vi "MBmaster.vi_tom.vi"(0 "Register address (0)":u16 max=247 format="%.0x", 1 "Modbus address (1)":u8=1 max=247, 2 "port number":i32, 5 "No. of points (1)":u16 max=247, 7 "Setpoints (0)":dbl[](array[numeric]) max=247.0 format="%.2f", 9 "Set digitals":bool[](array[boolean]), 11 "error in (no error)":errorcluster, 12 "Decimal points (0)":u8[](array[numeric]) max=4, 13 "ModBus Function":T1(ring)=enum."03 Read output registers") -> (4 "String send to device":string, 6 "String received from device":string, 8 "Process values":dbl[](array[numeric]) max=247.0 format="%.2f", 10 "Digitals read":bool[](array[boolean]), 15 "error out":errorcluster)   [LabVIEW 2010]
doc: "VI let you communicatie via a serial inerface with Modbus instruments.\n\nPS. No error checking is done in this version; Error clusters only implemented for future use - Users might implement this for their own needs...\n\nThis VI is referenced to the Modicon Modbus Protocol as described in the Modicon Modbus Protocol Reference Guide PI-MBUS-300 rev. D\n\nThis VI is only tested with a Eurotherm T103 unit controller but should alse work with any other Modbus Instrument.\n\nMaarten van Bree\nAIR technical automation, the Netherlands\n\nmvbree@euronet.nl\ninfo@air.nl\nhttp://www.air.nl"
panel:
  out "Calculated CRC":u16 format="%.0x"
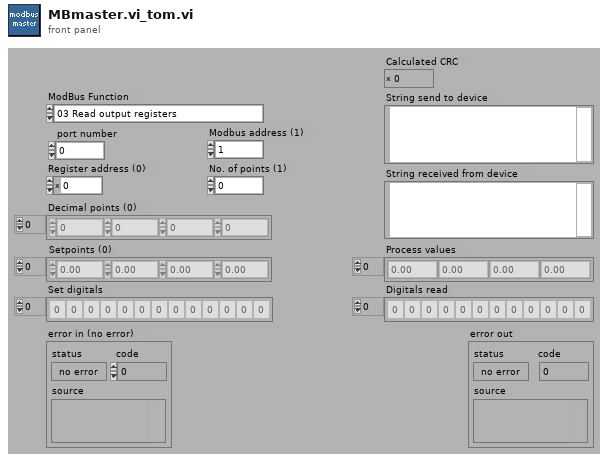
[diagram p1: front panel]
types:
  T1 = enum16{"01 Read digital output status", "02 Read digital input status", "03 Read output registers", "04 Read input registers", "05 Write single digital output", "06 Write single output register", "15 Write multiple digital outputs", "16 Write multiple output registers"}
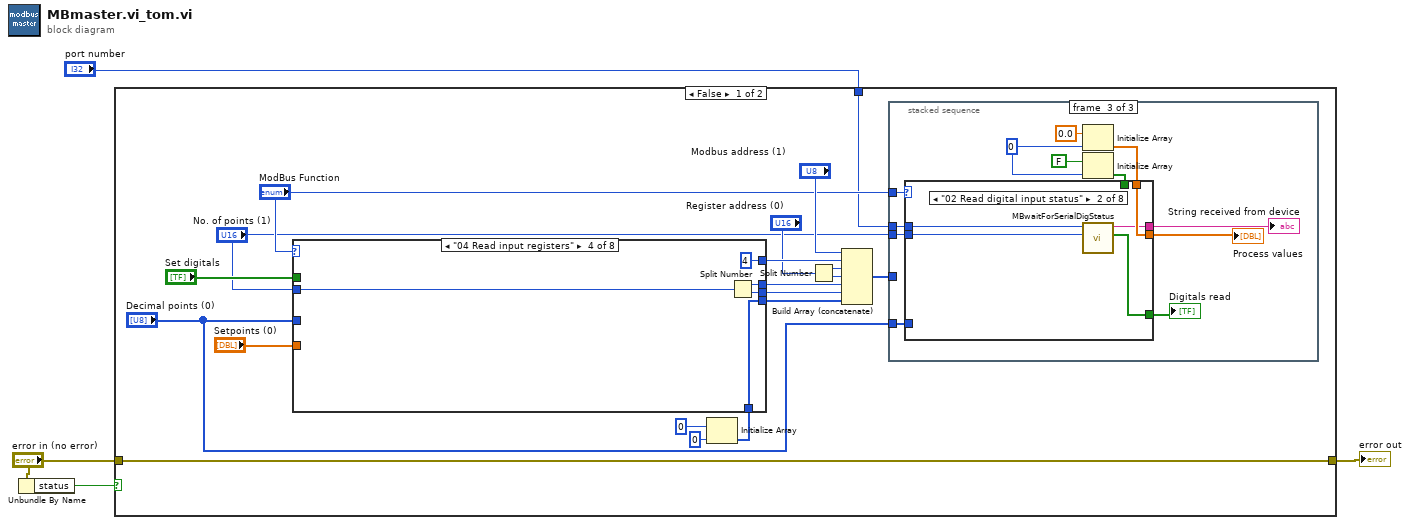
[diagram p0: block diagram]
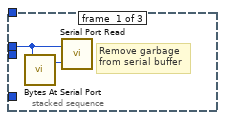
[diagram p2: hidden frame]
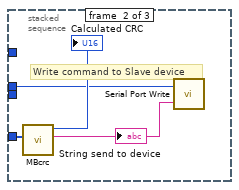
[diagram p3: hidden frame]
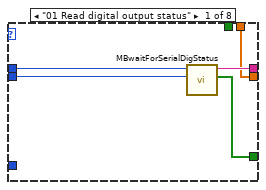
[diagram p4: hidden frame]
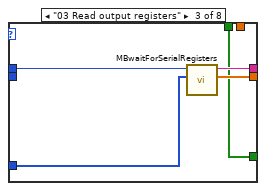
[diagram p5: hidden frame]
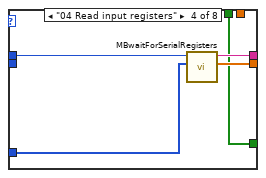
[diagram p6: hidden frame]
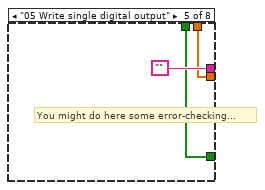
[diagram p7: hidden frame]
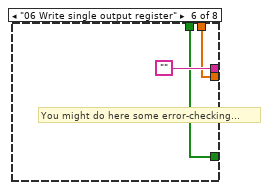
[diagram p8: hidden frame]
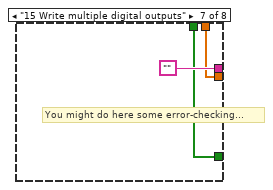
[diagram p9: hidden frame]
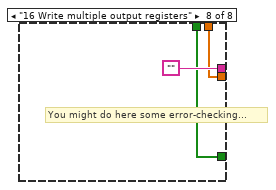
[diagram p10: hidden frame]
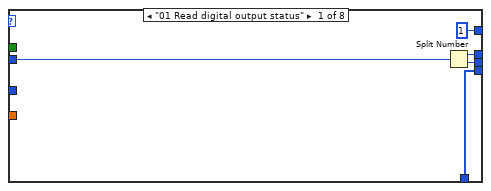
[diagram p11: hidden frame]
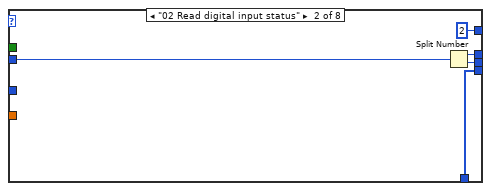
[diagram p12: hidden frame]
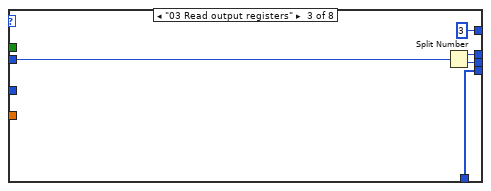
[diagram p13: hidden frame]
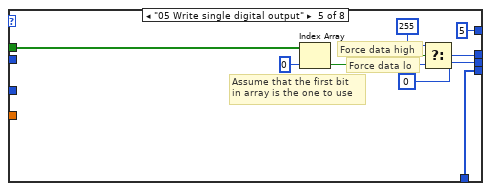
[diagram p14: hidden frame]
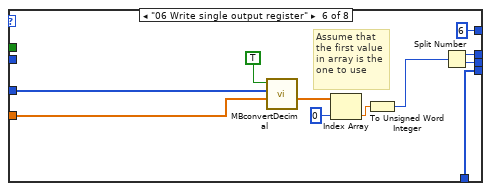
[diagram p15: hidden frame]
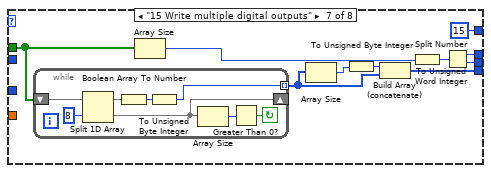
[diagram p16: hidden frame]
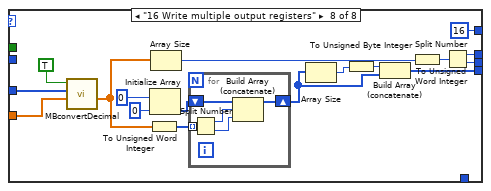
[diagram p17: hidden frame]
diagram:
  n1 = Unbundle By Name("error in (no error)") -> ("status"=w3:bool)
  n2 = case shown="False" w3 {
    tunnel: [w23 w153] -> w2
    tunnel: "error in (no error)" -> [w23 w153]
    tunnel: "port number" -> [w6 _]
    frame False {
      n3 = Initialize Array(u8 0, 0) -> (w7:u8[])
      n4 = case shown="\"04 Read input registers\"" "ModBus Function" {
        tunnel: "No. of points (1)" -> [w77 w82 w85 w90 _ _ _ _]
        tunnel: [u8 1 u8 2 u8 3 u8 4 u8 5 u8 6 u8 15 u8 16] -> w21
        tunnel: [w76 w81 w87 w92 w96 w105 w121 w141] -> w17
        tunnel: [w75 w80 w86 w91 w95 w104 w120 w142] -> w16
        tunnel: "Set digitals" -> [_ _ _ _ w100 _ w114 _]
        tunnel: "Setpoints (0)" -> [_ _ _ _ _ w111 _ w138]
        tunnel: "Decimal points (0)" -> [_ _ _ _ _ w110 _ w139]
        tunnel: [w74 w79 w84 w89 w94 w102 w118 w143] -> w10
        tunnel: w7 -> [w74 w79 w84 w89 w94 w102 _ _]
        frame "01 Read digital output status" {
          n5 = Split Number(x=w77) -> (hi(x)=w76:u8, lo(x)=w75:u8)
        }
        frame "02 Read digital input status" {
          n6 = Split Number(x=w82) -> (hi(x)=w81:u8, lo(x)=w80:u8)
        }
        frame "03 Read output registers" {
          n7 = Split Number(x=w85) -> (hi(x)=w87:u8, lo(x)=w86:u8)
        }
        frame "04 Read input registers" {
          n8 = Split Number(x=w90) -> (hi(x)=w92:u8, lo(x)=w91:u8)
        }
        frame "05 Write single digital output" {
          w95 = u8 0
          # "Force data lo"
          # "Force data high"
          # "Assume that the first bit\nin array is the one to use"
          n9 = Index Array(array=w100, index=0) -> (element=w98:bool)
          n10 = Select(t=u8 255, s=w98, f=w95) -> (s? t:f=w96:u8)
        }
        frame "06 Write single output register" {
          # "Assume that\nthe first value\nin array is the\none to use"
          n11 = call "MBconvertDecimal.vi"("Values"=w111, "Decimal points"=w110, "From (F) / to (T) decimal"=TRUE) -> ("New values"=w108:dbl[])  [unwired: 8 out]
          n12 = Index Array(array=w108, index=0) -> (element=w106:dbl)
          n13 = To Unsigned Word Integer(number=w106) -> (unsigned 16bit integer=w103:u16)
          n14 = Split Number(x=w103) -> (hi(x)=w105:u8, lo(x)=w104:u8)
        }
        frame "15 Write multiple digital outputs" {
          n15 = while {
            tunnel: [w123] -> w113 mode=indexing
            shift-left: w114 -> [w130]
            shift-right: [w128] -> _
            stop <- w126 continue-if-true
            n16 = Split 1D Array(array=w130, index=8 ("y")) -> (first subarray=w125:bool[], second subarray=w128:bool[])
            n17 = Boolean Array To Number(Boolean array=w125) -> (number=w124:u32)
            n18 = To Unsigned Byte Integer(number=w124) -> (unsigned 8bit integer=w123:u8)
            n19 = Array Size(array=w128) -> (size(s)=w127:i32)
            n20 = Greater Than 0?(x=w127) -> (x > 0?=w126:bool)
          }
          n21 = Array Size(array=w114) -> (size(s)=w115:i32)
          n22 = Array Size(array=w113) -> (size(s)=w117:i32)
          n23 = To Unsigned Byte Integer(number=w117) -> (unsigned 8bit integer=w116:u8)
          n24 = Build Array (concatenate)(w116, w113) -> (w118:u8[])
          n25 = To Unsigned Word Integer(number=w115) -> (unsigned 16bit integer=w119:u16)
          n26 = Split Number(x=w119) -> (hi(x)=w121:u8, lo(x)=w120:u8)
        }
        frame "16 Write multiple output registers" {
          n27 = call "MBconvertDecimal.vi"("Values"=w138, "Decimal points"=w139, "From (F) / to (T) decimal"=TRUE) -> ("New values"=w132:dbl[])  [unwired: 8 out]
          n28 = To Unsigned Word Integer(number=w132) -> (unsigned 16bit integer=w131:u16[])
          n29 = Initialize Array(u8 0, 0) -> (w134:u8[])
          n30 = Array Size(array=w132) -> (size(s)=w140:i32)
          n31 = for {
            shift-right: [w148] -> w133
            shift-left: w134 -> [w151]
            tunnel: w131 -> [w152] mode=indexing
            n32 = Split Number(x=w152) -> (hi(x)=w150:u8, lo(x)=w149:u8)
            n33 = Build Array (concatenate)(w151, w150, w149) -> (w148:u8[])
          }
          n34 = Array Size(array=w133) -> (size(s)=w145:i32)
          n35 = To Unsigned Byte Integer(number=w145) -> (unsigned 8bit integer=w144:u8)
          n36 = Build Array (concatenate)(w144, w133) -> (w143:u8[])
          n37 = To Unsigned Word Integer(number=w140) -> (unsigned 16bit integer=w146:u16)
          n38 = Split Number(x=w146) -> (hi(x)=w141:u8, lo(x)=w142:u8)
        }
      }
      n39 = Split Number(x="Register address (0)") -> (hi(x)=w19:u8, lo(x)=w18:u8)
      n40 = Build Array (concatenate)("Modbus address (1)", w21, w19, w18, w17, w16, w10) -> (w13:u8[])
      n41 = stacked-sequence {
        tunnel: w13 -> [_ w29 _]
        tunnel: w6 -> [w24 w27 w39]
        tunnel: "ModBus Function" -> [_ _ w41]
        tunnel: "Decimal points (0)" -> [_ _ w40]
        tunnel: "No. of points (1)" -> [_ _ w34]
        frame #0 {
          # "Remove garbage\nfrom serial buffer"
          n42 = call <vilib>:"Bytes At Serial Port.vi"("port number"=w24) -> ("byte count"=w25:u32)  [unwired: 1 out]
          n43 = call <vilib>:"Serial Port Read.vi"("requested byte count"=w25, "port number"=w24) -> ()  [unwired: 2 out]
        }
        frame #1 {
          # "Write command to Slave device"
          n44 = call "MBcrc.vi"("Data in:"=w29) -> ("Data out:"=w26:string, "CRC"=→"Calculated CRC":u16)  [unwired: 9 out]
          "String send to device" <- w26
          n45 = call <vilib>:"Serial Port Write.vi"("string to write"=w26, "port number"=w27) -> ()  [unwired: 1 out]
        }
        frame #2 {
          w33 = 0
          n46 = Initialize Array(0.0, w33) -> (w35:dbl[])
          n47 = Initialize Array(FALSE, w33) -> (w30:bool[])
          n48 = case shown="\"02 Read digital input status\"" w41 {
            tunnel: w40 -> [_ _ w55 w60 _ _ _ _]
            tunnel: w39 -> [w44 w48 w56 w61 _ _ _ _]
            tunnel: [w45 w51 w53 w59 w63 w66 w69 w72] -> w38
            tunnel: [w46 w50 w54 w58 "" "" "" ""] -> w37
            tunnel: w35 -> [w45 w51 _ _ w63 w66 w69 w72]
            tunnel: w34 -> [w43 w47 _ _ _ _ _ _]
            tunnel: [w42 w49 w52 w57 w62 w65 w68 w71] -> w31
            tunnel: w30 -> [_ _ w52 w57 w62 w65 w68 w71]
            frame "01 Read digital output status" {
              n49 = call "MBwaitForSerialDigStatus.vi"("No. of points(1)"=w43, "Serial port (0)"=w44) -> ("Digital status"=w42:bool[], "String read"=w46:string)  [unwired: 8 out]
            }
            frame "02 Read digital input status" {
              n50 = call "MBwaitForSerialDigStatus.vi"("No. of points(1)"=w47, "Serial port (0)"=w48) -> ("Digital status"=w49:bool[], "String read"=w50:string)  [unwired: 8 out]
            }
            frame "03 Read output registers" {
              n51 = call "MBwaitForSerialRegisters.vi"("Decimal points (0)"=w55, "Serial port (0)"=w56) -> ("Process values"=w53:dbl[], "String received from device"=w54:string)  [unwired: 2 in, 6 out]
            }
            frame "04 Read input registers" {
              n52 = call "MBwaitForSerialRegisters.vi"("Decimal points (0)"=w60, "Serial port (0)"=w61) -> ("Process values"=w59:dbl[], "String received from device"=w58:string)  [unwired: 2 in, 6 out]
            }
            frame "05 Write single digital output" {
              # "You might do here some error-checking..."
            }
            frame "06 Write single output register" {
              # "You might do here some error-checking..."
            }
            frame "15 Write multiple digital outputs" {
              # "You might do here some error-checking..."
            }
            frame "16 Write multiple output registers" {
              # "You might do here some error-checking..."
            }
          }
          "String received from device" <- w37
          "Process values" <- w38
          "Digitals read" <- w31
        }
      }
    }
    frame True {
    }
  }
  "error out" <- w2
